vi "Write Instrumentes to Use.vi"(10 "Instruments to Use":T1(array[cluster]), 11 "Test Framework in":refnum<class "Test Framework.lvclass">) -> (3 "Test Framework out":refnum<class "Test Framework.lvclass">)   [LabVIEW 2020, in "Test Framework.lvclass"]
uses:
  Test Framework.lvclass
  Instruments/Instrument.lvclass
  Test Framework.lvclass/Test Framework.ctl
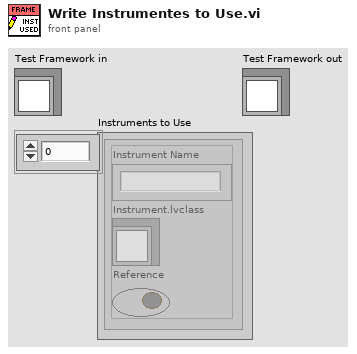
[diagram p1: front panel]
types:
  T1 = cluster{"Instrument Name":string, "Instrument.lvclass":refnum<class "Instrument.lvclass">, "Reference":bool}[]
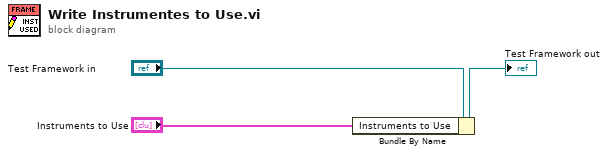
[diagram p0: block diagram]
diagram:
  n1 = Bundle By Name(cluster="Test Framework in", "Instruments to Use"="Instruments to Use") -> (→"Test Framework out":refnum<class "Test Framework.lvclass">)
